vi "Refresh SysCfg Session.vi"(6 "Timeout (180 s)":u32=180, 8 "error in (no error)":errorcluster, 11 "RT Management in":refnum<class "RT Management.lvclass">) -> (0 "error out":errorcluster, 3 "RT Management out":refnum<class "RT Management.lvclass">)   [LabVIEW 2015, in "RT Management.lvlib" / "RT Management.lvclass"]
uses:
  RT Management.lvclass
  SMI.lvlib
  <resource>/objmgr/nisysapi.rc
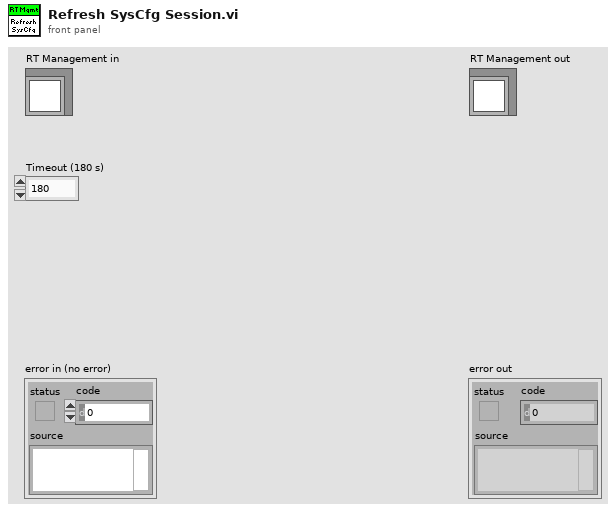
[diagram p1: front panel]
types:
  T1 = typedef "RT Management.lvlib/RT Management.lvclass/Status.ctl" = enum16{"Unknown", "Disconnected", "Running", "Unconfigured", "Install Mode", "No software installed", "Safe Mode (Corrupt Main Exe)", "Safe Mode (User Directed)", "Safe Mode (User Directed - Forced)", "Safe Mode (Software Error)", "Safe Mode (No Software Installed)", "Safe Mode (Corrupt Installation)", "Safe Mode (Improper Installation)", "Safe Mode (Main Program Not Found)", "Safe Mode (Software Update Required)", "Safe Mode (Unsupported RT Boot Partition)"}
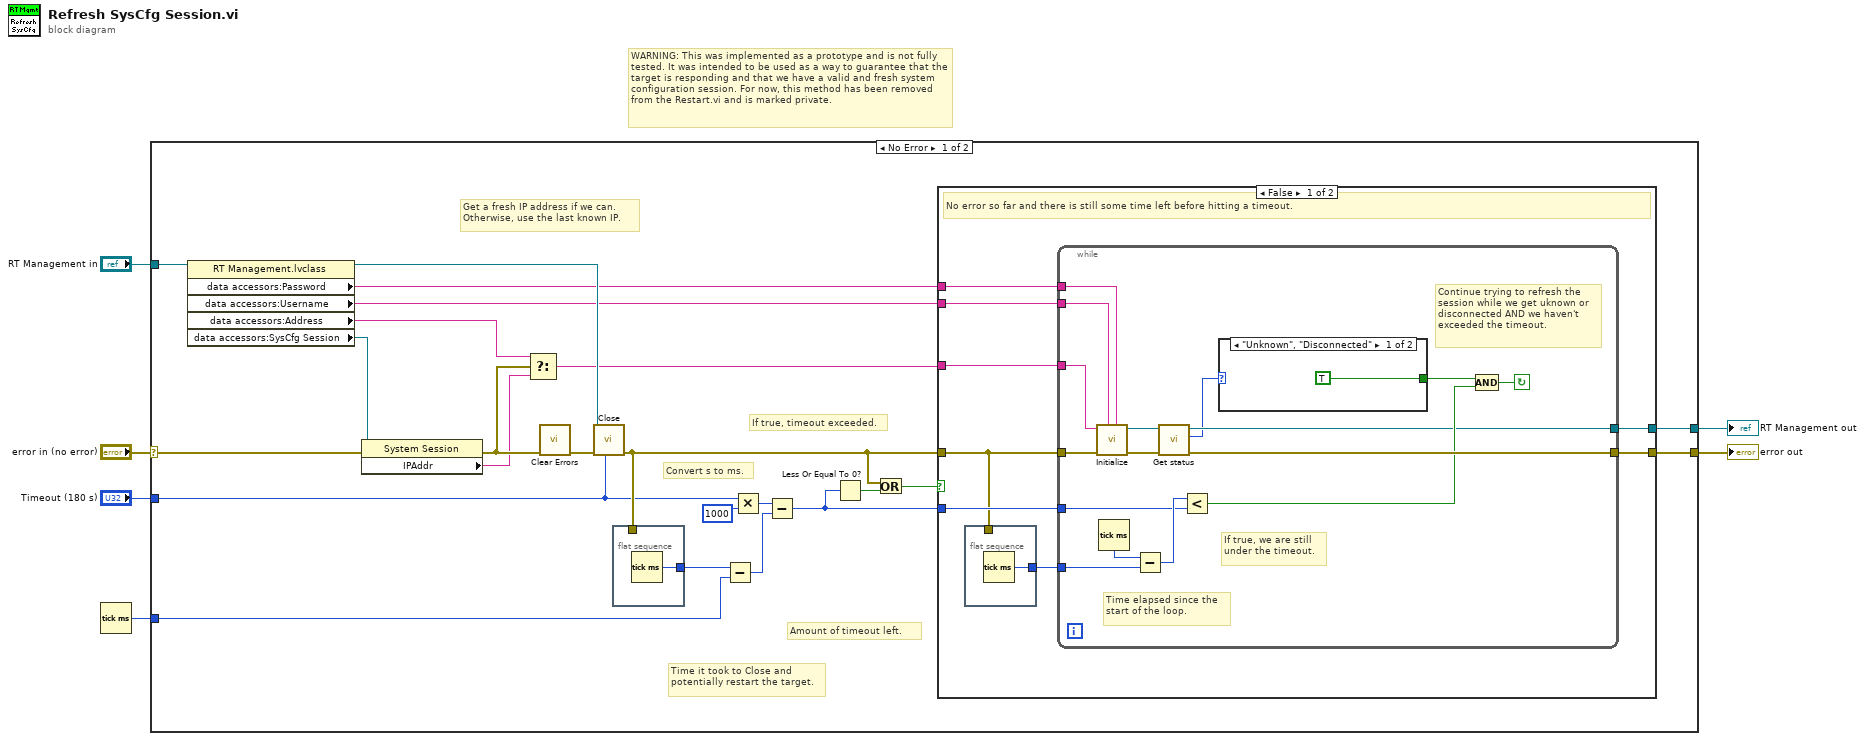
[diagram p0: block diagram]
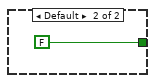
[diagram p2: hidden frame]
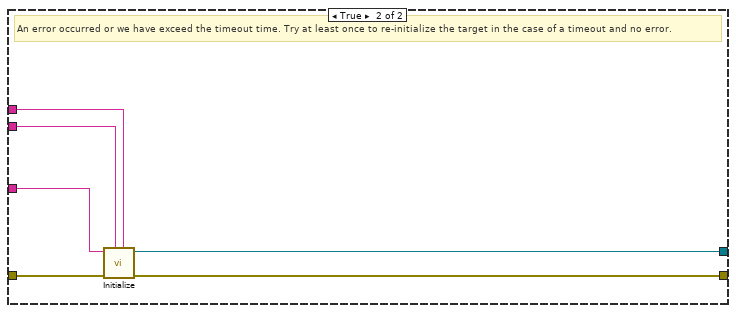
[diagram p3: hidden frame]
diagram:
  # "WARNING: This was implemented as a prototype and is not fully tested. It was intended to be used as a way to guarantee that the target is responding and that we have a valid and fresh system configuration session. For now, this method has been removed from the Restart.vi and is marked private."
  n1 = Tick Count (ms)() -> (millisecond timer value=w2:u32)
  n2 = case shown="No Error" "error in (no error)" {
    selector: "error in (no error)" -> [w26 w65]
    tunnel: [w11 w65] -> w5
    tunnel: [w10 w64] -> w3
    tunnel: "RT Management in" -> [w28 w64]
    tunnel: w2 -> [w18 _]
    tunnel: "Timeout (180 s)" -> [w7 _]
    frame No Error {
      # "Get a fresh IP address if we can. Otherwise, use the last known IP."
      # "Convert s to ms."
      # "If true, timeout exceeded."
      # "Amount of timeout left."
      # "Time it took to Close and potentially restart the target."
      n3 = property class="RT Management.lvclass"(reference=w28) -> (reference out=w22:refnum<class "RT Management.lvclass">, "data accessors:Password"=w19:string, "data accessors:Username"=w20:string, "data accessors:Address"=w25:string, "data accessors:SysCfg Session"=w27:refnum<k21>)  [unwired: 1 in, 1 out]
      n4 = property class="System Session"(reference=w27, error in=w26) -> (error out=w29:errorcluster, "IPAddr"=w24:string)  [unwired: 1 out]
      n5 = Select(t=w25, s=w29, f=w24) -> (s? t:f=w21:string)
      n6 = call <vilib>:"Clear Errors.vi"("error in (no error)"=w29) -> ("error out"=w23:errorcluster)  [unwired: 5 in, 1 out]
      n7 = call "Close.vi"("Timeout (180 s)"=w7, "error in (no error)"=w23, "RT Management in"=w22) -> ("error out"=w14:errorcluster)  [unwired: 8 in]
      n8 = flat-sequence {
        tunnel: w14 -> [_]
        tunnel: [w63] -> w12
        frame #0 {
          n9 = Tick Count (ms)() -> (millisecond timer value=w63:u32)
        }
      }
      n10 = Subtract(x=w12, y=w18) -> (x-y=w17:u32)
      n11 = Multiply(x=w7, y=u32 1000) -> (x*y=w9:u32)
      n12 = Subtract(x=w9, y=w17) -> (x-y=w16:u32)
      n13 = Less Or Equal To 0?(x=w16) -> (x <= 0?=w15:bool)
      n14 = Or(x=w14, y=w15) -> (x .or. y?=w13:bool)
      n15 = case shown="False" w13 {
        tunnel: w21 -> [w37 w61]
        tunnel: w20 -> [w36 w60]
        tunnel: w19 -> [w35 w59]
        tunnel: w14 -> [w33 w62]
        tunnel: w16 -> [w34 _]
        tunnel: [w31 w58] -> w11
        tunnel: [w30 w57] -> w10
        frame False {
          # "No error so far and there is still some time left before hitting a timeout."
          n16 = flat-sequence {
            tunnel: [w38] -> w32
            tunnel: w33 -> [_]
            frame #0 {
              n17 = Tick Count (ms)() -> (millisecond timer value=w38:u32)
            }
          }
          n18 = while {
            tunnel: w33 -> [w53]
            tunnel: w37 -> [w52]
            tunnel: w36 -> [w51]
            tunnel: w35 -> [w50]
            tunnel: w32 -> [w46]
            tunnel: w34 -> [w43]
            tunnel: [w54] -> w31
            tunnel: [w40] -> w30
            stop <- w41 continue-if-true
            # "If true, we are still under the timeout."
            # "Continue trying to refresh the session while we get uknown or disconnected AND we haven't exceeded the timeout."
            # "Time elapsed since the start of the loop."
            n19 = call "Initialize.vi"("Password"=w50, "Username (\"\" : target default)"=w51, "error in (no error)"=w53, "Target"=w52) -> ("error out"=w49:errorcluster, "RT Management out"=w48:refnum<class "RT Management.lvclass">)  [unwired: 5 in, 1 out]
            n20 = Tick Count (ms)() -> (millisecond timer value=w47:u32)
            n21 = Subtract(x=w47, y=w46) -> (x-y=w44:u32)
            n22 = call "Get status.vi"("error in (no error)"=w49, "RT Management in"=w48) -> ("error out"=w54:errorcluster, "Status"=w39:T1, "RT Management out"=w40:refnum<class "RT Management.lvclass">)  [unwired: 6 in, 1 out]
            n23 = Less?(x=w44, y=w43) -> (x < y?=w45:bool)
            n24 = case shown="\"Unknown\", \"Disconnected\"" w39 {
              tunnel: [TRUE FALSE] -> w42
              frame "Unknown", "Disconnected" {
              }
              frame Default {
              }
            }
            n25 = Compound Arithmetic op=AND(w42, w45) -> (w41:bool)
          }
        }
        frame True {
          # "An error occurred or we have exceed the timeout time. Try at least once to re-initialize the target in the case of a timeout and no error."
          n26 = call "Initialize.vi"("Password"=w59, "Username (\"\" : target default)"=w60, "error in (no error)"=w62, "Target"=w61) -> ("error out"=w58:errorcluster, "RT Management out"=w57:refnum<class "RT Management.lvclass">)  [unwired: 5 in, 1 out]
        }
      }
    }
    frame Error {
    }
  }
  "error out" <- w5
  "RT Management out" <- w3
